vi "Close.vi"(8 "error in (no error)":errorcluster, 11 "AI Ref In":T1) -> (0 "error out":errorcluster)   [LabVIEW 2021, in "AI.lvlib"]
doc: "Closes the reference to one or more analog input channels."
uses:
  <vilib>/myRIO/Instrument Drivers/Onboard IO/AI/AI.lvlib
  <vilib>/myRIO/Instrument Drivers/Onboard IO/AI/typedefs/AI Reference.ctl
  <vilib>/myRIO/Common/Instrument Driver Framework/Utilities/typedefs/myRIO Generic Hardware Reference.ctl
  <vilib>/myRIO/Common/Instrument Driver Framework/Utilities/typedefs/Hardware Version Enum.ctl
  <vilib>/myRIO/Common/Instrument Driver Framework/Utilities/typedefs/myRIO v1.0 Reference.ctl
  <vilib>/myRIO/Common/Instrument Driver Framework/Utilities/typedefs/Generic FPGA Reference.ctl
  <vilib>/myRIO/Common/Instrument Driver Framework/myRIO v1.0/AI/typedefs/AI Channels List.ctl
  <vilib>/myRIO/Common/Instrument Driver Framework/myRIO v1.0/AI/typedefs/AI Channels Enum.ctl
  <vilib>/myRIO/Common/Instrument Driver Framework/Utilities/typedefs/Analog Scaling Constants List.ctl
  <vilib>/myRIO/Common/Instrument Driver Framework/Utilities/typedefs/Analog Scaling Constants.ctl
  <vilib>/myRIO/Common/Instrument Driver Framework/myRIO v1.0/AI/vis/myRIO v1.0 Unreserve AI.vi
  <vilib>/myRIO/Common/Instrument Driver Framework/roboRIO v1.0/AI/vis/roboRIO v1.0 Unreserve AI.vi
  <vilib>/myRIO/Common/Instrument Driver Framework/ELVIS III v1.0/AI/vis/ELVIS III v1.0 Unreserve AI.vi
  <vilib>/myRIO/Common/Instrument Driver Framework/myRIO v1.0/Resource Manager/vis/myRIO v1.0 Unreserve Channel List.vi
  <vilib>/myRIO/Common/Instrument Driver Framework/myRIO v1.0/AI/vis/myRIO v1.0 Build MUX Configuration AI.vi
  <vilib>/myRIO/Common/Instrument Driver Framework/roboRIO v1.0/Resource Manager/vis/roboRIO v1.0 Unreserve Channel List.vi
  <vilib>/myRIO/Common/Instrument Driver Framework/roboRIO v1.0/AI/vis/roboRIO v1.0 Build MUX Configuration AI.vi
  <vilib>/myRIO/Common/Instrument Driver Framework/ELVIS III v1.0/AI/vis/ELVIS III v1.0 Build MUX Configuration AI.vi
  <vilib>/myRIO/Common/Instrument Driver Framework/myRIO v1.0/Resource Manager/vis/myRIO v1.0 Unreserve Channel.vi
  <vilib>/myRIO/Common/Instrument Driver Framework/roboRIO v1.0/Resource Manager/vis/roboRIO v1.0 Unreserve Channel.vi
  <vilib>/myRIO/Common/Instrument Driver Framework/myRIO v1.0/Resource Manager/vis/myRIO v1.0 Build Mutex Name.vi
  <vilib>/myRIO/Common/Instrument Driver Framework/roboRIO v1.0/Resource Manager/vis/roboRIO v1.0 Build Mutex Name.vi
  <vilib>/myRIO/Common/Instrument Driver Framework/Utilities/vis/Configuration Manager.vi
  <vilib>/myRIO/Common/Instrument Driver Framework/Utilities/vis/IO Manager.vi
  <vilib>/myRIO/Common/Instrument Driver Framework/ELVIS III v1.0/Resource Manager/vis/ELVIS III v1.0 Unreserve Channel List.vi
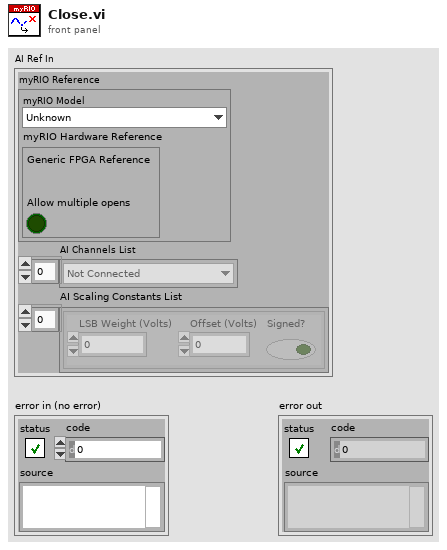
[diagram p1: front panel]
types:
  T1 = typedef "AI.lvlib/AI Reference.ctl" = cluster{"myRIO Reference":T2, "AI Channels List":T6, "AI Scaling Constants List":T8}
  T2 = typedef "myRIO Generic Hardware Reference.ctl" = cluster{"myRIO Model":T3, "myRIO Hardware Reference":T4}
  T3 = typedef "Hardware Version Enum.ctl" = enum16{"Unknown", "myRIO-1900", "myRIO-1950", "roboRIO", "NI ELVIS RIO CM", "ELVIS III"}
  T4 = typedef "myRIO v1.0 Reference.ctl" = cluster{"Generic FPGA Reference":T5, "Allow multiple opens":bool}
  T5 = typedef "Generic FPGA Reference.ctl" = refnum<k20>
  T6 = typedef "AI Channels List.ctl" = T7[]
  T7 = typedef "AI Channels Enum.ctl" = enum16{"Not Connected", "AudioIn/Left", "AudioIn/Right", "C/AI0", "C/AI1", "A/AI0", "A/AI1", "A/AI2", "A/AI3", "A/AI4", "A/AI5", "A/AI6", "A/AI7", "B/AI0", "B/AI1", "B/AI2", "B/AI3", "B/AI4", "B/AI5", "B/AI6", "B/AI7", "AI/AI0", "AI/AI1", "AI/AI2", "AI/AI3", "A/AI0 (DIFF)", "A/AI1 (DIFF)", "A/AI2 (DIFF)", "A/AI3 (DIFF)", "B/AI0 (DIFF)", "B/AI1 (DIFF)", "B/AI2 (DIFF)", "B/AI3 (DIFF)"}
  T8 = typedef "Analog Scaling Constants List.ctl" = T9[]
  T9 = typedef "Analog Scaling Constants.ctl" = cluster{"LSB Weight (Volts)":dbl, "Offset (Volts)":dbl, "Signed?":bool}
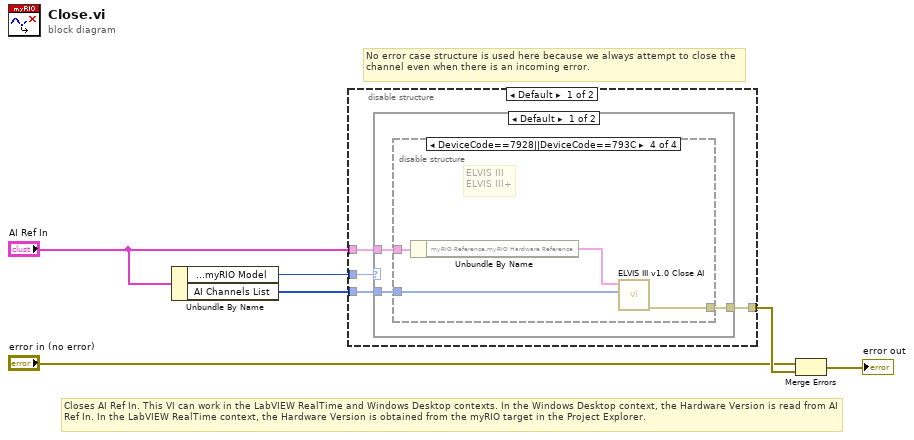
[diagram p0: block diagram]
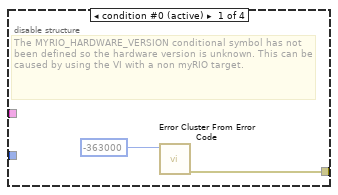
[diagram p2: hidden frame]
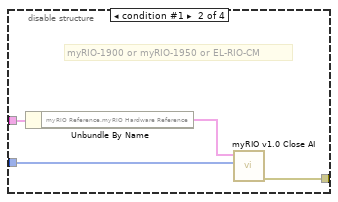
[diagram p3: hidden frame]
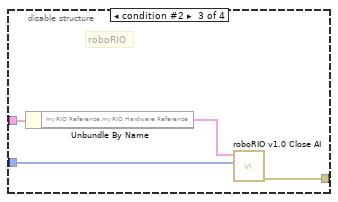
[diagram p4: hidden frame]
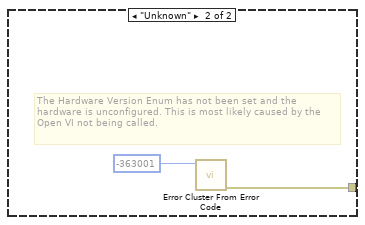
[diagram p5: hidden frame]
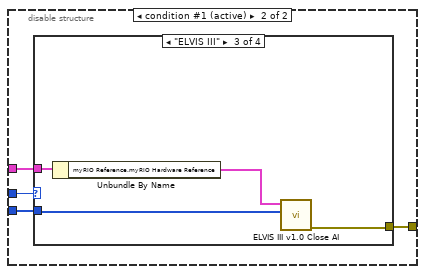
[diagram p6: hidden frame]
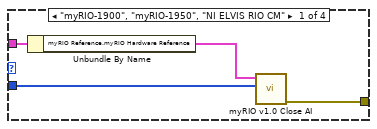
[diagram p7: hidden frame]
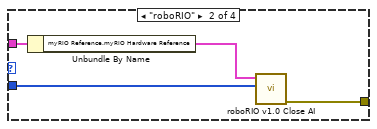
[diagram p8: hidden frame]
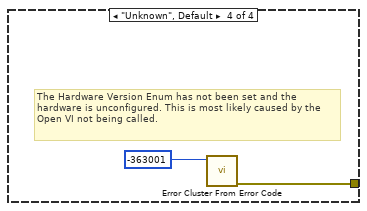
[diagram p9: hidden frame]
diagram:
  # "No error case structure is used here because we always attempt to close the channel even when there is an incoming error."
  # "Closes AI Ref In. This VI can work in the LabVIEW RealTime and Windows Desktop contexts. In the Windows Desktop context, the Hardware Version is read from AI Ref In. In the LabVIEW RealTime context, the Hardware Version is obtained from the myRIO target in the Project Explorer."
  n1 = Unbundle By Name("AI Ref In") -> ("myRIO Reference.myRIO Model"=w2:T3, "AI Channels List"=w1:T6)
  n2 = disable-structure shown="Default" {
    disable-tunnel: "AI Ref In" -> [w10 w32]
    disable-tunnel: [w9 w33] -> w6
    disable-tunnel: w2 -> [w8 w31]
    disable-tunnel: w1 -> [w7 w30]
    frame condition #0 {
      n3 = case shown="Default" w8 {
        tunnel: w10 -> [w13 _]
        tunnel: [w12 w28] -> w9
        tunnel: w7 -> [w11 _]
        frame Default {
          n4 = disable-structure shown="DeviceCode==7928||DeviceCode==793C" {
            disable-tunnel: w13 -> [_ w19 w23 w26]
            disable-tunnel: [w14 w18 w22 w24] -> w12
            disable-tunnel: w11 -> [_ w16 w20 w25]
            frame condition #0 (active) {
              # "The MYRIO_HARDWARE_VERSION conditional symbol has not been defined so the hardware version is unknown. This can be caused by using the VI with a non myRIO target."
              n5 = call <vilib>:"Error Cluster From Error Code.vi"("error code (0)"=-363000) -> ("error out"=w14:errorcluster)  [unwired: 8 in]
            }
            frame condition #1 {
              # "myRIO-1900 or myRIO-1950 or EL-RIO-CM"
              n6 = Unbundle By Name(w19) -> ("myRIO Reference.myRIO Hardware Reference"=w17:T4)
              n7 = call <vilib>:"myRIO v1.0 Close AI.vi"("AI Channel List"=w16, "myRIO Ref In"=w17) -> ("error out"=w18:errorcluster)  [unwired: 9 in]
            }
            frame condition #2 {
              # "roboRIO"
              n8 = Unbundle By Name(w23) -> ("myRIO Reference.myRIO Hardware Reference"=w21:T4)
              n9 = call <vilib>:"roboRIO v1.0 Close AI.vi"("AI Channel List"=w20, "myRIO Ref In"=w21) -> ("error out"=w22:errorcluster)  [unwired: 9 in]
            }
            frame condition #3 {
              # "ELVIS III\nELVIS III+"
              n10 = Unbundle By Name(w26) -> ("myRIO Reference.myRIO Hardware Reference"=w27:T4)
              n11 = call <vilib>:"ELVIS III v1.0 Close AI.vi"("AI Channel List"=w25, "myRIO Ref In"=w27) -> ("error out"=w24:errorcluster)  [unwired: 9 in]
            }
          }
        }
        frame "Unknown" {
          # "The Hardware Version Enum has not been set and the hardware is unconfigured. This is most likely caused by the Open VI not being called."
          n12 = call <vilib>:"Error Cluster From Error Code.vi"("error code (0)"=-363001) -> ("error out"=w28:errorcluster)  [unwired: 8 in]
        }
      }
    }
    frame condition #1 (active) {
      n13 = case shown="\"ELVIS III\"" w31 {
        tunnel: w32 -> [w37 w41 w44 _]
        tunnel: [w36 w40 w42 w46] -> w33
        tunnel: w30 -> [w34 w38 w43 _]
        frame "myRIO-1900", "myRIO-1950", "NI ELVIS RIO CM" {
          n14 = Unbundle By Name(w37) -> ("myRIO Reference.myRIO Hardware Reference"=w35:T4)
          n15 = call <vilib>:"myRIO v1.0 Close AI.vi"("AI Channel List"=w34, "myRIO Ref In"=w35) -> ("error out"=w36:errorcluster)  [unwired: 9 in]
        }
        frame "roboRIO" {
          n16 = Unbundle By Name(w41) -> ("myRIO Reference.myRIO Hardware Reference"=w39:T4)
          n17 = call <vilib>:"roboRIO v1.0 Close AI.vi"("AI Channel List"=w38, "myRIO Ref In"=w39) -> ("error out"=w40:errorcluster)  [unwired: 9 in]
        }
        frame "ELVIS III" {
          n18 = Unbundle By Name(w44) -> ("myRIO Reference.myRIO Hardware Reference"=w45:T4)
          n19 = call <vilib>:"ELVIS III v1.0 Close AI.vi"("AI Channel List"=w43, "myRIO Ref In"=w45) -> ("error out"=w42:errorcluster)  [unwired: 9 in]
        }
        frame "Unknown", Default {
          # "The Hardware Version Enum has not been set and the hardware is unconfigured. This is most likely caused by the Open VI not being called."
          n20 = call <vilib>:"Error Cluster From Error Code.vi"("error code (0)"=-363001) -> ("error out"=w46:errorcluster)  [unwired: 8 in]
        }
      }
    }
  }
  n21 = Merge Errors("error in (no error)", w6) -> (→"error out":errorcluster)
